vi "action.vi"(0 "HGF_Device_ErrorQuery":refnum<class "HGF_Device_ErrorQuery.lvclass">, 2 "HGF_Visitable":refnum<class "HGF_Visitable.lvclass">, 5 "error in (no error)":errorcluster) -> (14 "dup HGF_Device_ErrorQuery":refnum<class "HGF_Device_ErrorQuery.lvclass">, 16 "dup HGF_Visitable":refnum<class "HGF_Visitable.lvclass">, 19 "error out":errorcluster)   [LabVIEW 2014, in "HGF_DeviceBaseClasses.lvlib" / "HGF_Device_ErrorQuery.lvclass"]
doc: "This is a dynamic dispatch VI that is called from Visitor.visit(). It will call member VIs of Visitable to perform the requested action which means: calling public methods of Visitable child class.\n\n<B>Hint:</B> This method is abstract and need to be implemented by child classes."
uses:
  HGF_Device_ErrorQuery.lvclass
  HGF_DeviceBase/HGF_DeviceBase.lvclass
  HGF_BaseClasses/HGF_Visitable/HGF_Visitable.lvclass
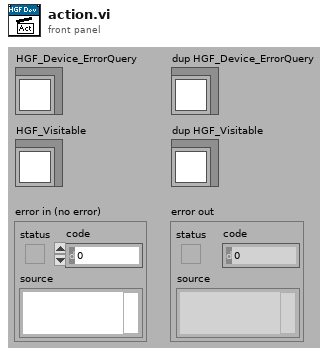
[diagram p1: front panel]
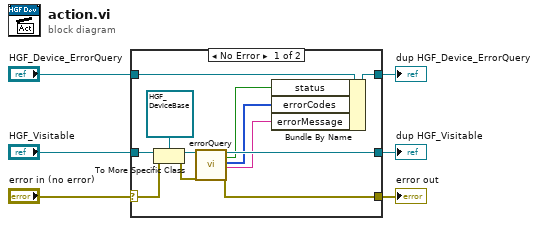
[diagram p0: block diagram]
diagram:
  n1 = case shown="No Error" "error in (no error)" {
    selector: "error in (no error)" -> [w16 w20]
    tunnel: "HGF_Visitable" -> [w18 w21]
    tunnel: [w12 w21] -> w5
    tunnel: [w7 w20] -> w3
    tunnel: [w14 w19] -> w1
    tunnel: "HGF_Device_ErrorQuery" -> [w15 w19]
    frame No Error {
      n2 = To More Specific Class(target class=refnum<class "HGF_DeviceBase.lvclass"> refnum ("HGF_DeviceBaseClasses.lvlib:HGF_DeviceBase.lvclass"), reference=w18, error in=w16) -> (specific class reference=w13:refnum<class "HGF_DeviceBase.lvclass">, error out=w11:errorcluster)
      n3 = call-dynamic "errorQuery.vi"("HGF_DeviceBase"=w13, "error in (no error)"=w11) -> ("dup HGF_DeviceBase"=w12:refnum<class "HGF_DeviceBase.lvclass">, "status"=w10:bool, "errorCodes"=w9:i32[], "errorMessage"=w8:string, "error out"=w7:errorcluster)  [unwired: 13 out]
      n4 = Bundle By Name(cluster=w15, "status"=w10, "errorCodes"=w9, "errorMessage"=w8) -> (w14:refnum<class "HGF_Device_ErrorQuery.lvclass">)
    }
    frame Error {
    }
  }
  "error out" <- w3
  "dup HGF_Device_ErrorQuery" <- w1
  "dup HGF_Visitable" <- w5
